vi "aal_Complex Modulator with Phase.vi"   [LabVIEW 2020, in "NI_AAL_SigProc.lvlib"]
uses:
  <vilib>/Analysis/NI_AAL_SigProc.lvlib
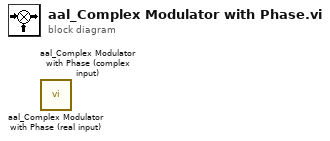
[diagram p0: block diagram]
diagram:
  n1 = call <vilib>:"aal_Complex Modulator with Phase (real input).vi"() -> ()  [unwired: 11 in, 1 out]
  n2 = call <vilib>:"aal_Complex Modulator with Phase (complex input).vi"() -> ()  [unwired: 11 in, 1 out]
